vi "Remove by Index.vi"(8 "error in (no error)":errorcluster, 10 "Index":i32, 11 "Config Manager in":refnum<class "Config Manager.lvclass">) -> (0 "error out":errorcluster, 3 "Config Manager out":refnum<class "Config Manager.lvclass">)   [LabVIEW 2020, in "CDM-Config.lvlib" / "Config Manager.lvclass"]
uses:
  Config Manager.lvclass
  Config Manager.lvclass/Config Manager.ctl
  Config Element/Config Element.lvclass
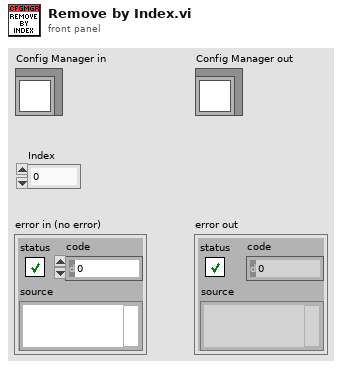
[diagram p1: front panel]
types:
  T1 = typedef "CDM-Config.lvlib/Config Manager.lvclass/Ref Data.ctl" = cluster{"Elements":refnum<class "Config Element.lvclass">[], "Hierarchy Map":map{string[], i32}, "Element Map":map{refnum<class "Config Element.lvclass">, i32}}
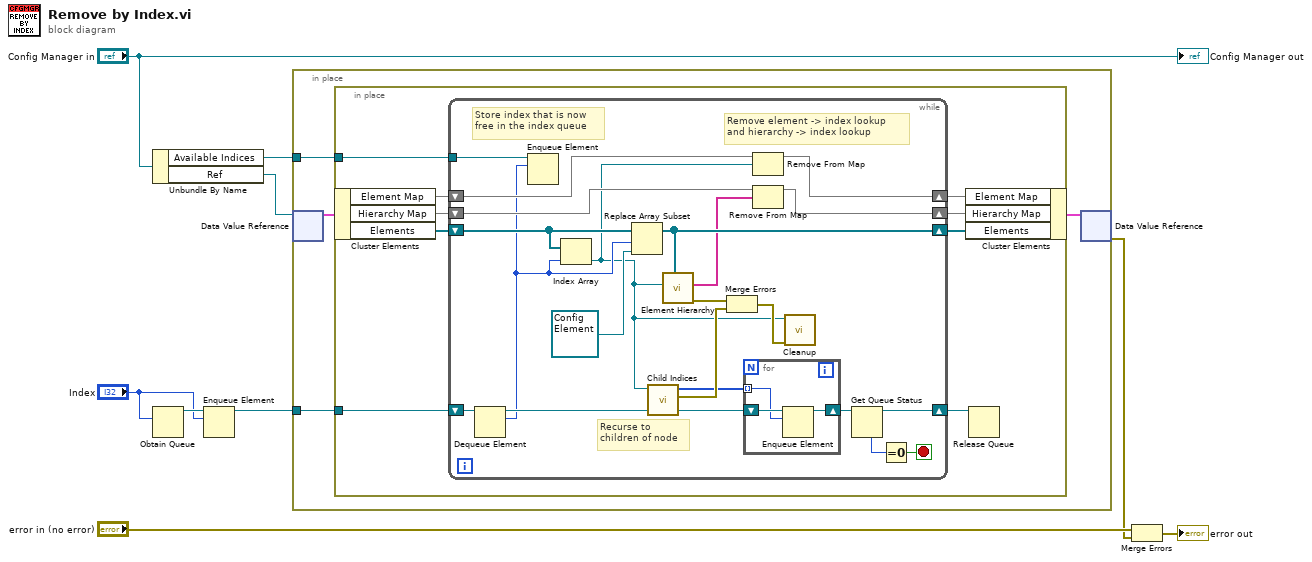
[diagram p0: block diagram]
diagram:
  n1 = Unbundle By Name("Config Manager in") -> ("Available Indices"=w1:refnum<queue>, "Ref"=w8:refnum<data-value>)
  n2 = Obtain Queue(element data type="Index") -> (queue out=w4:refnum<queue>)  [unwired: 4 in, 2 out]
  n3 = Enqueue Element(queue=w4, element="Index") -> (queue out=w2:refnum<queue>)  [unwired: 2 in, 2 out]
  n4 = in-place {
    in-place-border: w2 -> [w11]
    in-place-border: w1 -> [w10]
    n5 = in-place-dvr #1(w8) -> (w13:T1)  [unwired: 1 out]
    n6 = in-place {
      in-place-border: w11 -> [w16]
      in-place-border: w10 -> [w15]
      n7 = in-place-cluster #2(w13) -> ("Element Map"=w18:map{refnum<class "Config Element.lvclass">, i32}, "Hierarchy Map"=w22:map{string[], i32}, "Elements"=w21:refnum<class "Config Element.lvclass">[])
      n8 = while {
        shift-right: [w39] -> w19
        shift-left: w22 -> [w41]
        shift-right: [w26] -> w20
        shift-left: w21 -> [w40]
        shift-right: [w37] -> w17
        shift-left: w18 -> [w38]
        shift-right: [w35] -> w14
        shift-left: w16 -> [w36]
        tunnel: w15 -> [w28]
        stop <- w33 stop-if-true
        # "Recurse to children of node"
        # "Remove element -> index lookup\nand hierarchy -> index lookup"
        # "Store index that is now free in the index queue"
        n9 = Dequeue Element(queue=w36) -> (queue out=w31:refnum<queue>, element=w27:i32)  [unwired: 2 in, 2 out]
        n10 = Enqueue Element(queue=w28, element=w27) -> ()  [unwired: 2 in, 3 out]
        n11 = Index Array(array=w40, index=w27) -> (element=w24:refnum<class "Config Element.lvclass">)
        n12 = Replace Array Subset(array=w40, new element=refnum<class "Config Element.lvclass"> refnum ("new element/subarray"), index=w27) -> (w26:refnum<class "Config Element.lvclass">[])
        n13 = call "Child Indices.vi"("Config Element in"=w24) -> ("error out"=w42:errorcluster, "Children"=w30:i32[])  [unwired: 9 in]
        n14 = call "Element Hierarchy.vi"("Elements"=w26, "Config Element in"=w24) -> ("error out"=w25:errorcluster, "Hierarchy"=w23:string[])  [unwired: 8 in]
        n15 = Merge Errors(w25, w42) -> (w43:errorcluster)
        n16 = for {
          shift-right: [w44] -> w29
          shift-left: w31 -> [w46]
          tunnel: w30 -> [w45] mode=indexing
          n17 = Enqueue Element(queue=w46, element=w45) -> (queue out=w44:refnum<queue>)  [unwired: 2 in, 2 out]
        }
        n18 = Remove From Map(10:w24, 11:w38) -> (3:w37:map{refnum<class "Config Element.lvclass">, i32})  [unwired: 2 out]
        n19 = Remove From Map(10:w23, 11:w41) -> (3:w39:map{string[], i32})  [unwired: 2 out]
        n20 = call "Cleanup.vi"("error in (no error)"=w43, "Config Element in"=w24) -> ()  [unwired: 9 in, 1 out]
        n21 = Get Queue Status(queue=w29) -> (queue out=w35:refnum<queue>, # elements in queue=w34:i32)  [unwired: 2 in, 6 out]
        n22 = Equal To 0?(x=w34) -> (x = 0?=w33:bool)
      }
      n23 = in-place-cluster #2("Element Map"=w17, "Hierarchy Map"=w19, "Elements"=w20) -> (w12:T1)
      n24 = Release Queue(queue=w14) -> ()  [unwired: 2 in, 3 out]
    }
    n25 = in-place-dvr #1(w12) -> (w5:errorcluster)  [unwired: 1 out]
  }
  n26 = Merge Errors("error in (no error)", w5) -> (→"error out":errorcluster)
  "Config Manager out" <- "Config Manager in"
